vi "fft.vi"() -> ()   [LabVIEW 2015]
uses:
  <vilib>/Analysis/2dsp.llb/Real FFT.vi
  <vilib>/Analysis/NI_AALBase.lvlib
  <vilib>/Analysis/NI_AALPro.lvlib
panel:
  out "载波信号":cluster{dbl, dbl, "sine wave":dbl[]}(graph)
  in  "cycles 2":dbl
  in  "sample of freq 2":dbl
  in  "cycle of freq 2":dbl
  in  "phase in 2":dbl format="%0.2f"
  in  "amplitude 2":dbl=1.0 format="%0.2f"
  out "appended array":i32[](array[numeric])
  in  "stop":bool
  out "Waveform Graph 2":cluster{dbl, dbl, "sine wave":dbl[]}(graph)
  in  "FFT size":i32=-1
  in  "shift?":bool
  out "基带信号":cluster{dbl, dbl, "sine wave":dbl[]}(graph)
  in  "cycles":dbl
  in  "sample of freq":dbl
  in  "cycle of freq":dbl
  in  "phase in":dbl format="%0.2f"
  in  "amplitude":dbl=1.0 format="%0.2f"
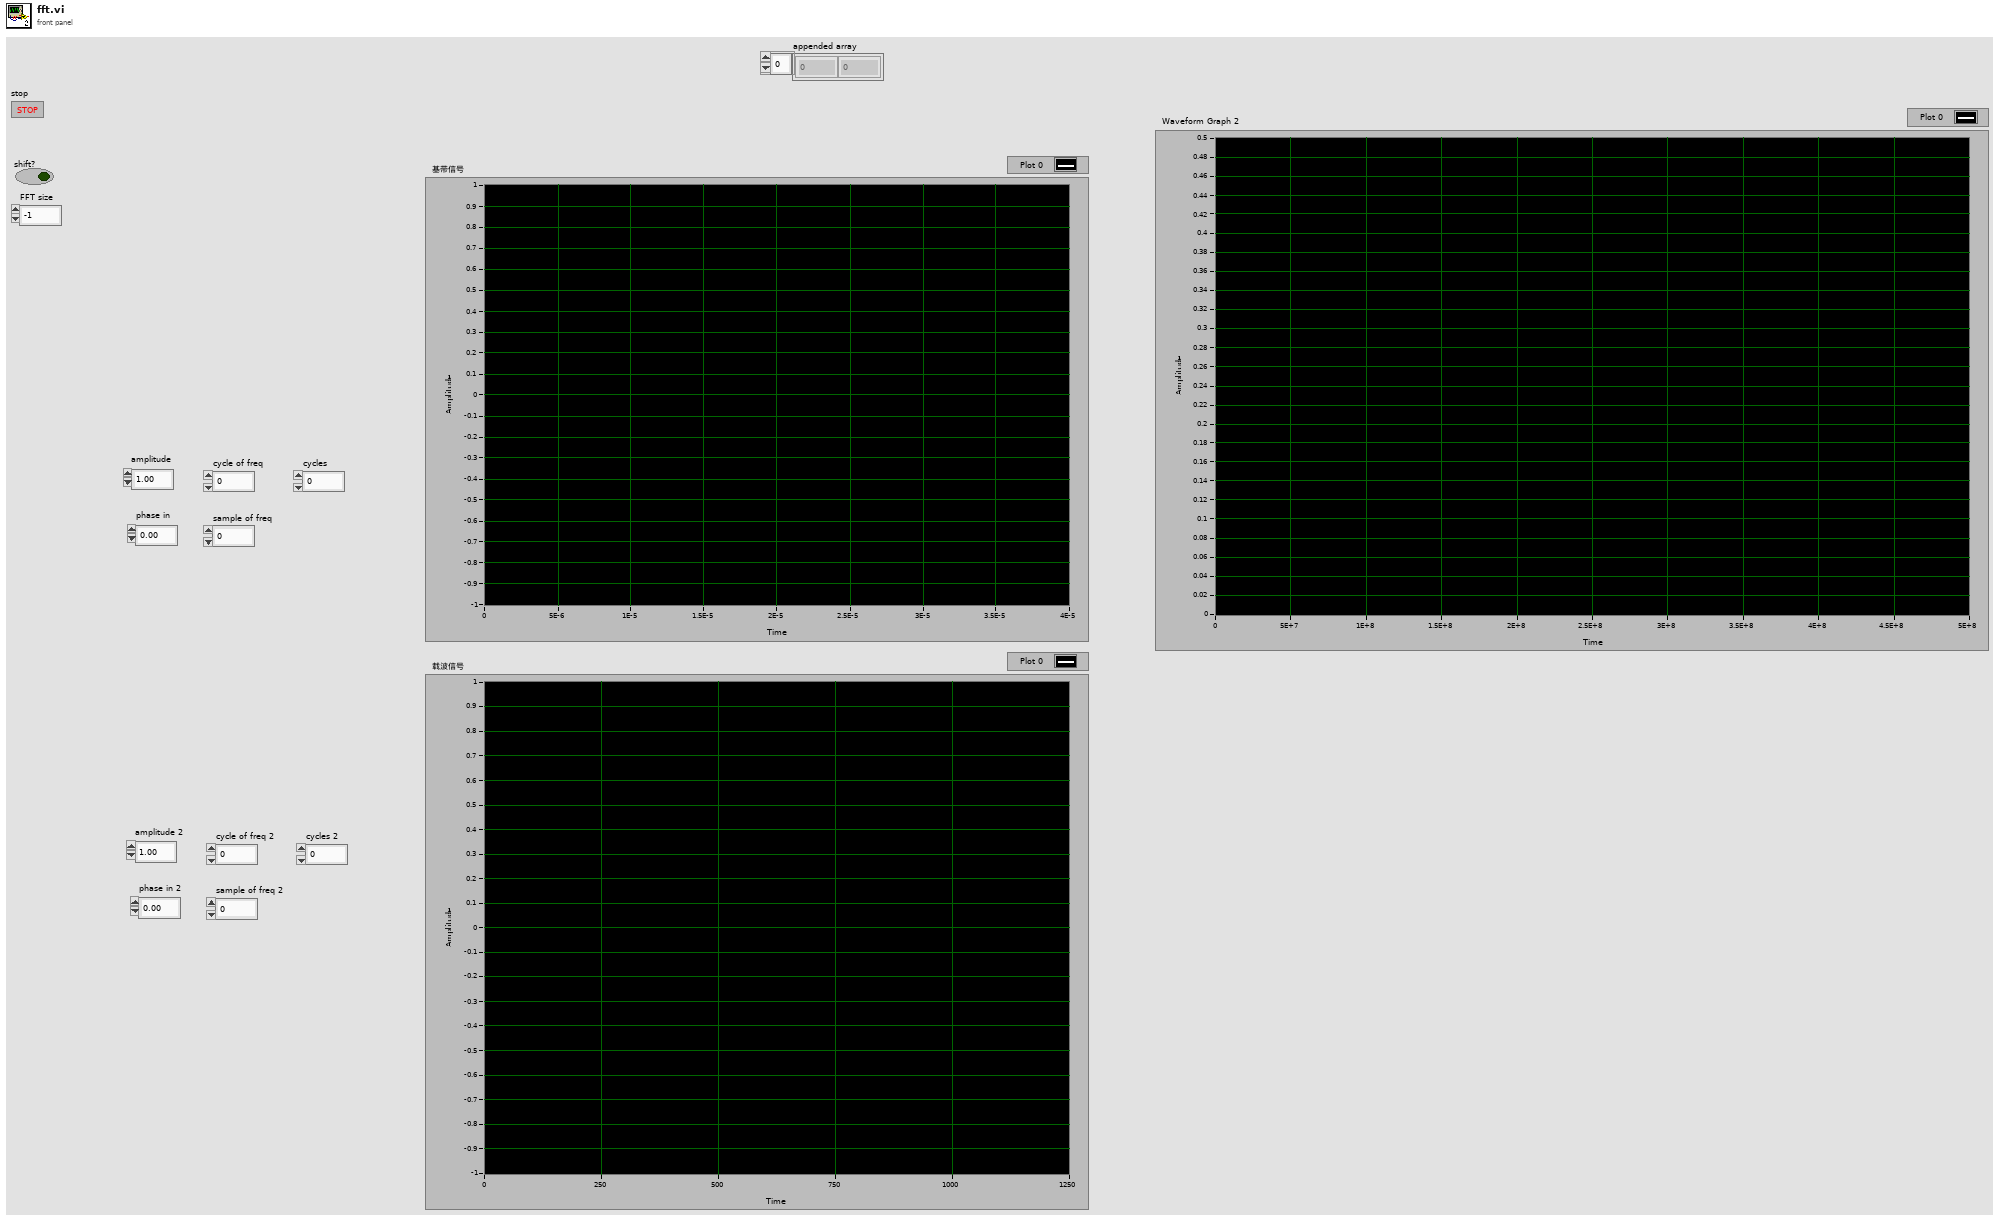
[diagram p1: front panel]
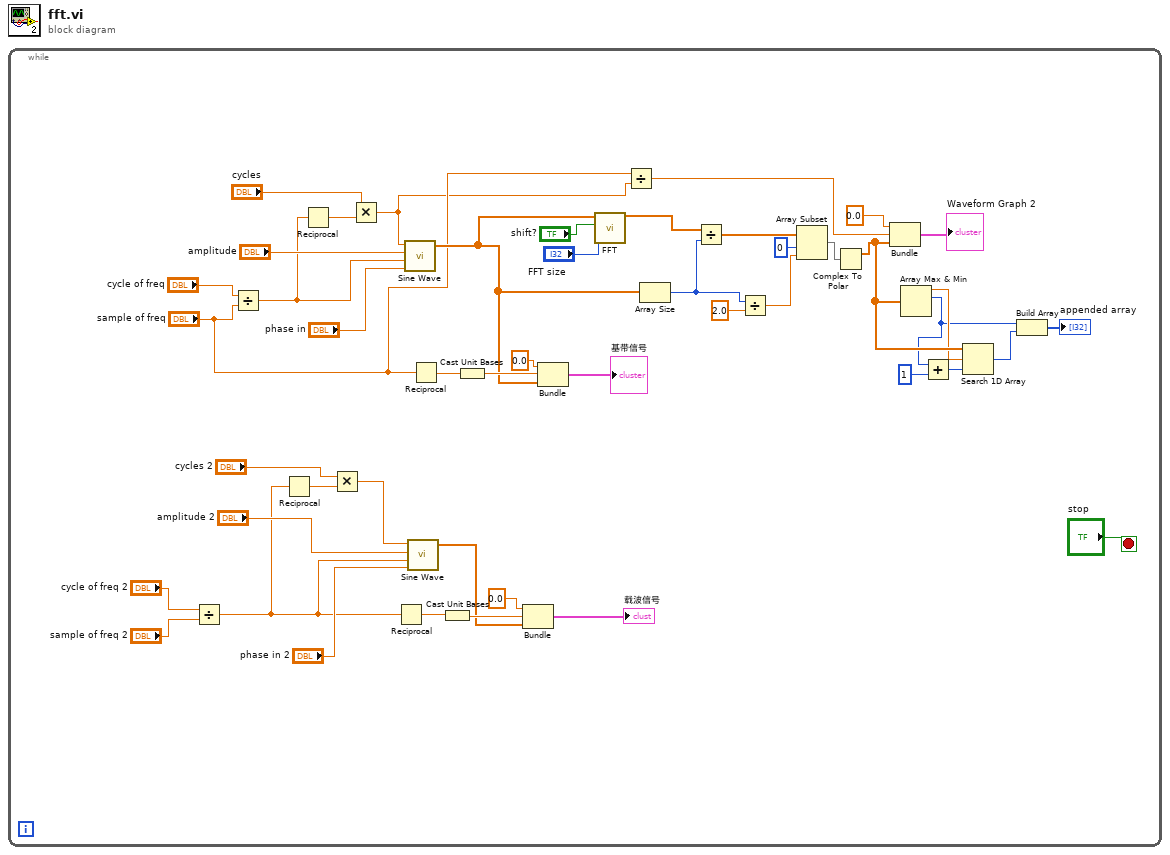
[diagram p0: block diagram]
diagram:
  n1 = while {
    stop <- "stop" stop-if-true
    n2 = Divide(x="cycle of freq 2", y="sample of freq 2") -> (x/y=w6:dbl)
    n3 = Divide(x="cycle of freq", y="sample of freq") -> (x/y=w42:dbl)
    n4 = Reciprocal(x=w6) -> (1/x=w10:dbl)
    n5 = Reciprocal(x=w42) -> (1/x=w43:dbl)
    n6 = Multiply(x="cycles 2", y=w10) -> (x*y=w8:dbl)
    n7 = Multiply(x="cycles", y=w43) -> (x*y=w26:dbl)
    n8 = Reciprocal(x=w6) -> (1/x=w5:dbl)
    n9 = call <vilib>:"Sine Wave.vi"("samples"=w26, "amplitude"="amplitude", "frequency"=w42, "phase in"="phase in") -> ("sine wave"=w34:dbl[])  [unwired: 1 in, 2 out]
    n10 = call <vilib>:"Sine Wave.vi"("samples"=w8, "amplitude"="amplitude 2", "frequency"=w6, "phase in"="phase in 2") -> ("sine wave"=w2:dbl[])  [unwired: 1 in, 2 out]
    n11 = Reciprocal(x="sample of freq") -> (1/x=w40:dbl)
    n12 = Cast Unit Bases(0:w5) -> (2:w4:dbl)  [unwired: 1 in]
    n13 = Cast Unit Bases(0:w40) -> (2:w39:dbl)  [unwired: 1 in]
    n14 = Bundle(0.0, w4, "sine wave"=w2) -> (→"载波信号":cluster{dbl, dbl, "sine wave":dbl[]})  [unwired: 1 in]
    n15 = Bundle(0.0, w39, "sine wave"=w34) -> (→"基带信号":cluster{dbl, dbl, "sine wave":dbl[]})  [unwired: 1 in]
    n16 = call-poly <vilib>:"FFT.vi"("FFT size"="FFT size", "shift?"="shift?", "X"=w34) -> ("FFT {X}"=w33:cdb[])  [unwired: 7 in, 1 out]
    n17 = Divide(x="sample of freq", y=w26) -> (x/y=w28:dbl)
    n18 = Array Size(array=w34) -> (size(s)=w30:i32)
    n19 = Divide(x=w33, y=w30) -> (x/y=w32:cdb[])
    n20 = Divide(x=w30, y=2.0) -> (x/y=w29:dbl)
    n21 = Array Subset(array=w32, index=0, length=w29) -> (w21:cdb[])
    n22 = Complex To Polar(r * e^(i*theta)=w21) -> (r=w20:dbl[])  [unwired: 1 out]
    n23 = Bundle(0.0, w28, w20) -> (→"Waveform Graph 2":cluster{dbl, dbl, dbl[]})  [unwired: 1 in]
    n24 = Array Max & Min(array=w20) -> (max value=w16:dbl, max index (indices)=w15:i32)  [unwired: 2 out]
    n25 = Add(x=w15, y=1) -> (x+y=w19:i32)
    n26 = Search 1D Array(1D array=w20, element=w16, start index (0)=w19) -> (index of element=w17:i32)
    n27 = Build Array(w15, w17) -> (→"appended array":i32[])
  }
